vi "Get Data from SLSC.vi"(8 "error in (no error)":errorcluster, 10 "SLSC NVMEM Session In":refnum<class "SLSC Interface.lvclass">, 11 "SLSC Switch in":refnum<class "SLSC Switch.lvclass">) -> (0 "error out":errorcluster, 2 "SLSC NVMEM Session Out":refnum<class "SLSC Interface.lvclass">, 3 "SLSC Switch out":refnum<class "SLSC Switch.lvclass">)   [LabVIEW 2015, in "SLSC Switch.lvlib" / "SLSC Switch.lvclass"]
uses:
  SLSC Switch.lvclass
  <vilib>/National Instruments/SLSC Local or Remote Interface/SLSC Interface Class/SLSC Interface.lvclass
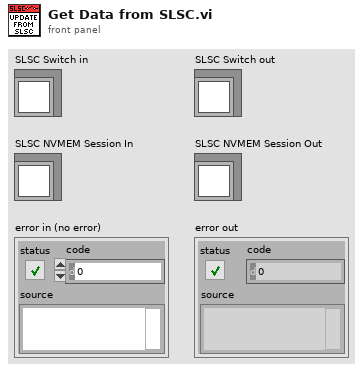
[diagram p1: front panel]
types:
  T1 = typedef "SLSC Switch.lvlib/SLSC Switch.lvclass/Topology.ctl" = cluster{"name":string, "InitialState":T2, "ChannelList":T3, "ConnectionList":T4[], "MuxList":cluster{"Src":string, "Dests":string[]}[]}
  T2 = typedef "SLSC Switch.lvlib/SLSC Switch.lvclass/JSON.InitialState.ctl" = cluster{"Open":string[], "Close":string[]}
  T3 = typedef "SLSC Switch.lvlib/SLSC Switch.lvclass/JSON.ChannelList.ctl" = cluster{"Names":string[]}
  T4 = typedef "SLSC Switch.lvlib/SLSC Switch.lvclass/JSON.ConnectionList.ctl" = cluster{"Src":string, "Dest":string, "Relays":string[]}
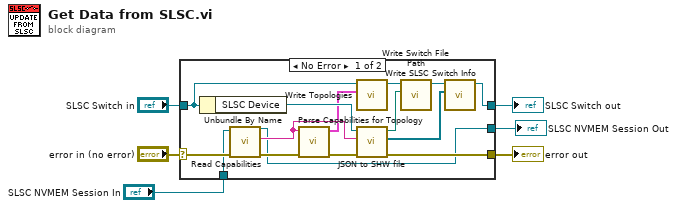
[diagram p0: block diagram]
diagram:
  n1 = case shown="No Error" "error in (no error)" {
    selector: "error in (no error)" -> [w16 w24]
    tunnel: [w20 w24] -> w5
    tunnel: "SLSC Switch in" -> [w15 w23]
    tunnel: [w14 w23] -> w3
    tunnel: "SLSC NVMEM Session In" -> [w8 w22]
    tunnel: [w7 w22] -> w1
    frame No Error {
      n2 = Unbundle By Name(w15) -> ("SLSC Device"=w13:refnum<k21>)
      n3 = call "Read Capabilities.vi"("error in (no error)"=w16, "SLSC NVMEM Session In"=w8) -> ("error out"=w10:errorcluster, "capabilities"=w12:string, "SLSC NVMEM Session Out"=w7:refnum<class "SLSC Interface.lvclass">)  [unwired: 7 in]
      n4 = call "Parse Capabilities for Topology.vi"("error in (no error)"=w10, "Capabilities JSON In"=w12) -> ("error out"=w9:errorcluster, "Topology Info"=w11:T1[])  [unwired: 8 in]
      n5 = call "Write Topologies.vi"("Topologies in"=w11, "SLSC Switch in"=w15) -> ("SLSC Switch out"=w21:refnum<class "SLSC Switch.lvclass">)  [unwired: 9 in]
      n6 = call "JSON to SHW file.vi"("error in (no error)"=w9, "Capabilities JSON In"=w12, "device"=w13) -> ("error out"=w20:errorcluster, "SLSC Switch Info"=w17:refnum<class "Relay.lvclass">[], "SHW Path Out"=w18:path)  [unwired: 6 in]
      n7 = call "Write Switch File Path.vi"("Switch File Path"=w18, "SLSC Switch in"=w21) -> ("SLSC Switch out"=w19:refnum<class "SLSC Switch.lvclass">)  [unwired: 9 in]
      n8 = call "Write SLSC Switch Info.vi"("Relays In"=w17, "SLSC Switch in"=w19) -> ("SLSC Switch out"=w14:refnum<class "SLSC Switch.lvclass">)  [unwired: 9 in]
    }
    frame Error {
    }
  }
  "error out" <- w5
  "SLSC Switch out" <- w3
  "SLSC NVMEM Session Out" <- w1
